vi "pathrun.vi"(11 "时间格式字符串(%c)":string="PMdata") -> (2 "引用句柄输出":refnum<file>)   [LabVIEW 2018]
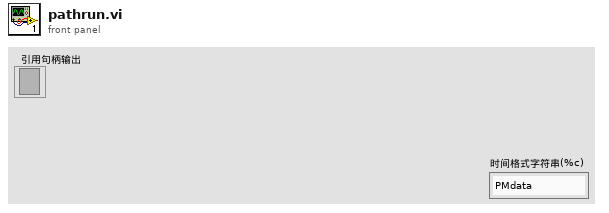
[diagram p1: front panel]
types:
  T1 = enum16{"open", "replace", "create", "open or create", "replace or create", "replace or create with confirmation"}
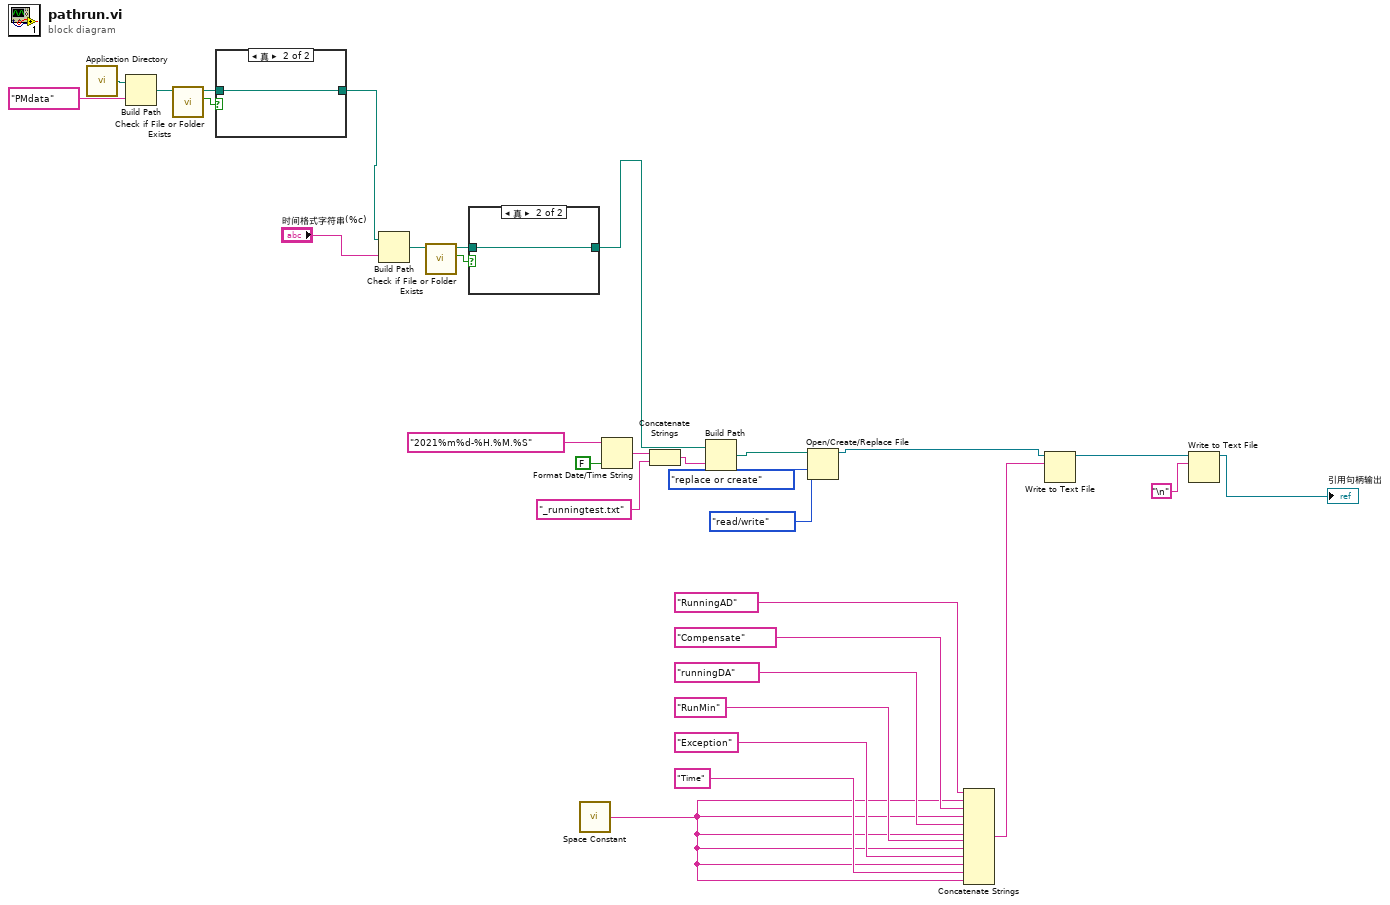
[diagram p0: block diagram]
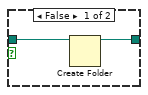
[diagram p2: hidden frame]
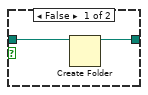
[diagram p3: hidden frame]
diagram:
  n1 = call <vilib>:"Application Directory.vi"() -> ("Application Directory"=w31:path)
  n2 = Build Path(base path=w31, name or relative path="PMdata" ("时间格式字符串(%c)")) -> (appended path=w29:path)
  n3 = call <vilib>:"Check if File or Folder Exists.vi"("path"=w29) -> ("file or folder exists?"=w28:bool, "dup path"=w27:path)  [unwired: 8 in, 1 out]
  n4 = case shown="真" w28 {
    tunnel: [w32 w34] -> w2
    tunnel: w27 -> [w33 w34]
    frame False {
      n5 = Create Folder(path (use dialog)=w33) -> (created path=w32:path)  [unwired: 2 in, 2 out]
    }
    frame True {
    }
  }
  n6 = Build Path(base path=w2, name or relative path="时间格式字符串(%c)") -> (appended path=w5:path)
  n7 = call <vilib>:"Check if File or Folder Exists.vi"("path"=w5) -> ("file or folder exists?"=w4:bool, "dup path"=w3:path)  [unwired: 8 in, 1 out]
  n8 = case shown="真" w4 {
    tunnel: [w35 w37] -> w1
    tunnel: w3 -> [w36 w37]
    frame False {
      n9 = Create Folder(path (use dialog)=w36) -> (created path=w35:path)  [unwired: 2 in, 2 out]
    }
    frame True {
    }
  }
  n10 = call <vilib>:"Space Constant.vi"() -> ("String"=w7:string)
  n11 = Format Date/Time String(time format string (%c)="2021%m%d-%H.%M.%S" ("时间格式字符串(%c)"), UTC format=FALSE ("UTC格式")) -> (date/time string=w24:string)  [unwired: 1 in]
  n12 = Concatenate Strings(w24, "_runningtest.txt" ("字符串")) -> (w22:string)
  n13 = Build Path(base path=w1, name or relative path=w22) -> (appended path=w26:path)
  n14 = Open/Create/Replace File(file path (use dialog)=w26, operation (0:open)=T1."replace or create" ("操作(0:open)"), access (0:read/write)=enum16{"read/write", "read-only", "write-only"}."read/write" ("权限(0:read/write)")) -> (refnum out=w10:refnum<file>)  [unwired: 3 in, 2 out]
  n15 = Concatenate Strings("RunningAD" ("字符串"), w7, "Compensate" ("字符串"), w7, "runningDA" ("字符串"), w7, "RunMin" ("字符串"), w7, "Exception" ("字符串"), w7, "Time" ("字符串"), w7) -> (w11:string)
  n16 = Write to Text File ("写入文本文件")(file (use dialog)=w10, text=w11) -> (refnum out=w17:refnum<file>)  [unwired: 2 in, 2 out]
  n17 = Write to Text File(file (use dialog)=w17, text="\n") -> (refnum out=→"引用句柄输出":refnum<file>)  [unwired: 2 in, 2 out]
